vi "PVCAM_CheckContStatus.vi"(8 "error in (no error)":errorcluster, 11 "hCam":i16) -> (0 "error out":errorcluster, 1 "buffer_cnt":u32, 2 "return type":i16, 3 "status":i16, 4 "bytes_cnt":u32)   [LabVIEW 2021]
uses:
  pvcam64.dll
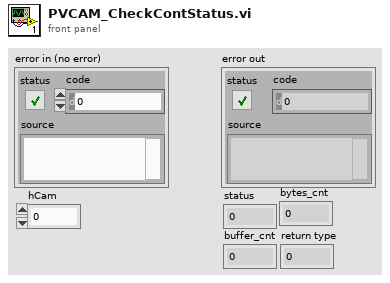
[diagram p1: front panel]
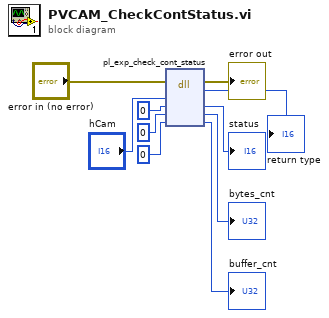
[diagram p0: block diagram]
diagram:
  n1 = dll-call lib="pvcam64.dll" fn="pl_exp_check_cont_status"(error in="error in (no error)", "hCam"="hCam", "status"=i16 0, "bytes_cnt"=u32 0 ("bytes_remaining"), "buffer_cnt"=u32 0) -> (error out=→"error out":errorcluster, "return type"=→"return type":i16, "status"=→"status":i16, "bytes_cnt"=→"bytes_cnt":u32, "buffer_cnt"=→"buffer_cnt":u32)  [unwired: 3 in, 1 out]
